vi "Setup Test.vi"() -> ()   [LabVIEW 2019, in "Menu Button.xctl"]
doc: "JSMA Module Template - Top Level UI 0.2.0.4\nRob Humfeld - Jet Engineering\nCopyright (c) 2019, Jet Engineering"
uses:
  Menu Button.xctl
  State 1.ctl
panel:
  out "Menu Config":variant
  in  "1st Run":bool
  out "Header":string
  in  "Radio Button":T1(radio)
  in  "Display State In":T2={"Header"="", "Label[]"=[], "DisableButtonsLUT"=variant(bool[] []), "Menu Config"=variant}
  in  "Path":path=path "C:/Projects/Emerson-PDLabUpdate-Codeline/Main Codeline/Software/Code/Shared/XControls/Menu Button/config/MenuConfig.ini"
  # "1. Drop the controls that make up the appearance\nof the XControl here.\n\n2. Resize the window to fit the controls\n\n3. If the XControl is of fixed size,  make the \n window not resizable from VI Properties->Window Appearance.\n\n4. If you want the controls to automatically size when the XControl sizes, check  \"Scale all objects on front panel when window resizes\" in File->VI Properties->Window Size page.\n\n5. Show the block diagram and handle events for the controls on this panel."
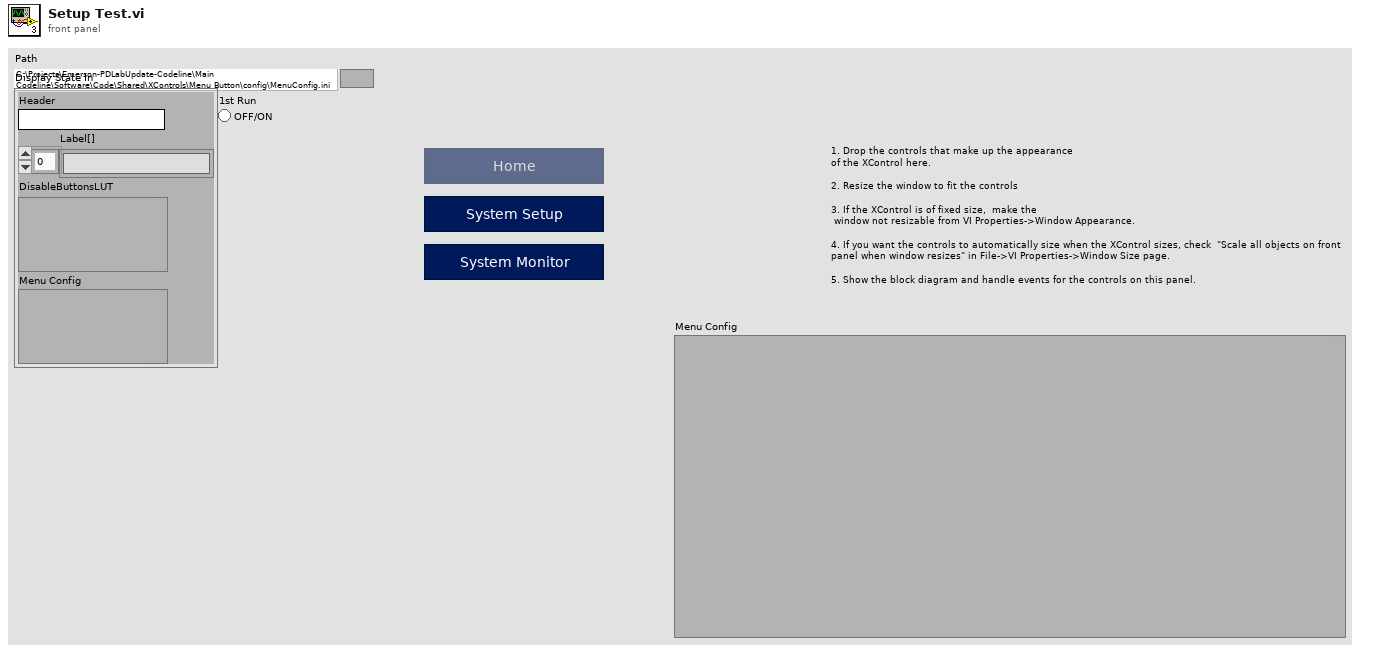
[diagram p1: front panel]
types:
  T1 = enum32{"No Selection", "System Setup", "System Monitor", "Test Selection", "Data Review", "Radio Selection 5", "Radio Selection 6", "Radio Selection 7", "Radio Selection 8", "Radio Selection 9", "Radio Selection 10"}
  T2 = typedef "Menu Button.xctl/State 1.ctl" = cluster{"Header":string, "Label[]":string[], "DisableButtonsLUT":variant, "Menu Config":variant}
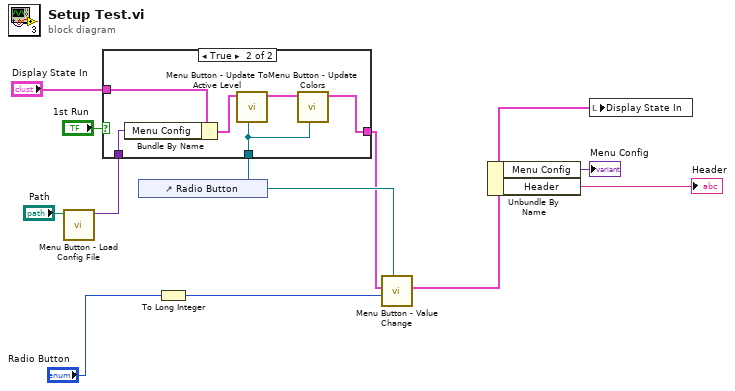
[diagram p0: block diagram]
diagram:
  n1 = call "Menu Button - Load Config File.vi"("Path"="Path") -> ("MenuConfig"=w9:variant)  [unwired: 7 in, 3 out]
  n2 = control-ref of="Radio Button"() -> (w4:refnum<vi>)
  n3 = case shown="True" "1st Run" {
    tunnel: "Display State In" -> [w12 w18]
    tunnel: w9 -> [_ w17]
    tunnel: [w12 w14] -> w1
    tunnel: w4 -> [_ w13]
    frame False {
    }
    frame True {
      n4 = Bundle By Name(cluster=w18, "Menu Config"=w17) -> (w16:T2)
      n5 = call "Menu Button - Update To Active Level.vi"("RadioButtonsControl in"=w13, "Display State In in"=w16) -> ("Display State In out"=w15:T2)  [unwired: 9 in]
      n6 = call "Menu Button - Update Colors.vi"("RadioButtonsControl in"=w13, "Display State In in"=w15) -> ("Display State In out"=w14:T2)  [unwired: 9 in]
    }
  }
  n7 = To Long Integer(number="Radio Button") -> (32bit integer=w6:i32)
  n8 = call "Menu Button - Value Change.vi"("RadioButtonsControl in"=w4, "Numeric"=w6, "Display State In in"=w1) -> ("Display State In out"=w2:T2)  [unwired: 7 in, 1 out]
  n9 = Unbundle By Name(w2) -> ("Menu Config"=→"Menu Config":variant, "Header"=→"Header":string)
  n10 = local write "Display State In"(w2) -> ()
